vi "CannonProjectileGameFramework.vi"() -> ()   [LabVIEW 2018]
panel:
  out "Distance":dbl
  out "?":cluster{dbl[], dbl[]}(graph)
  out "Score":dbl
  out "Attempt":i32
  out "Wind (mph)":dbl
  out "Target Distance (m)":dbl
  in  "?":bool
  in  "?":bool
  in  "Height (m)":dbl
  in  "Power":dbl
  in  "Angle (deg)":dbl
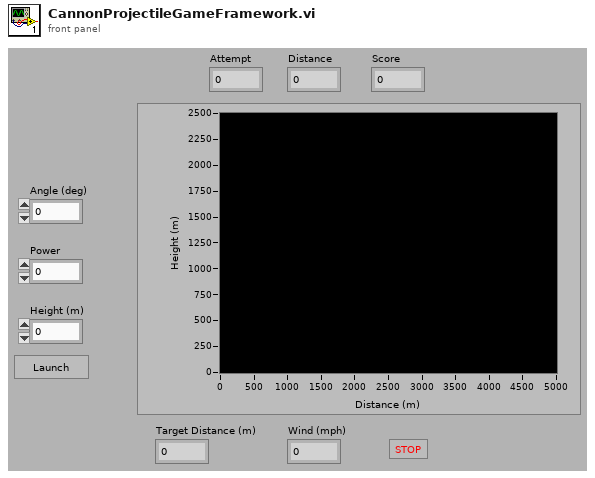
[diagram p1: front panel]
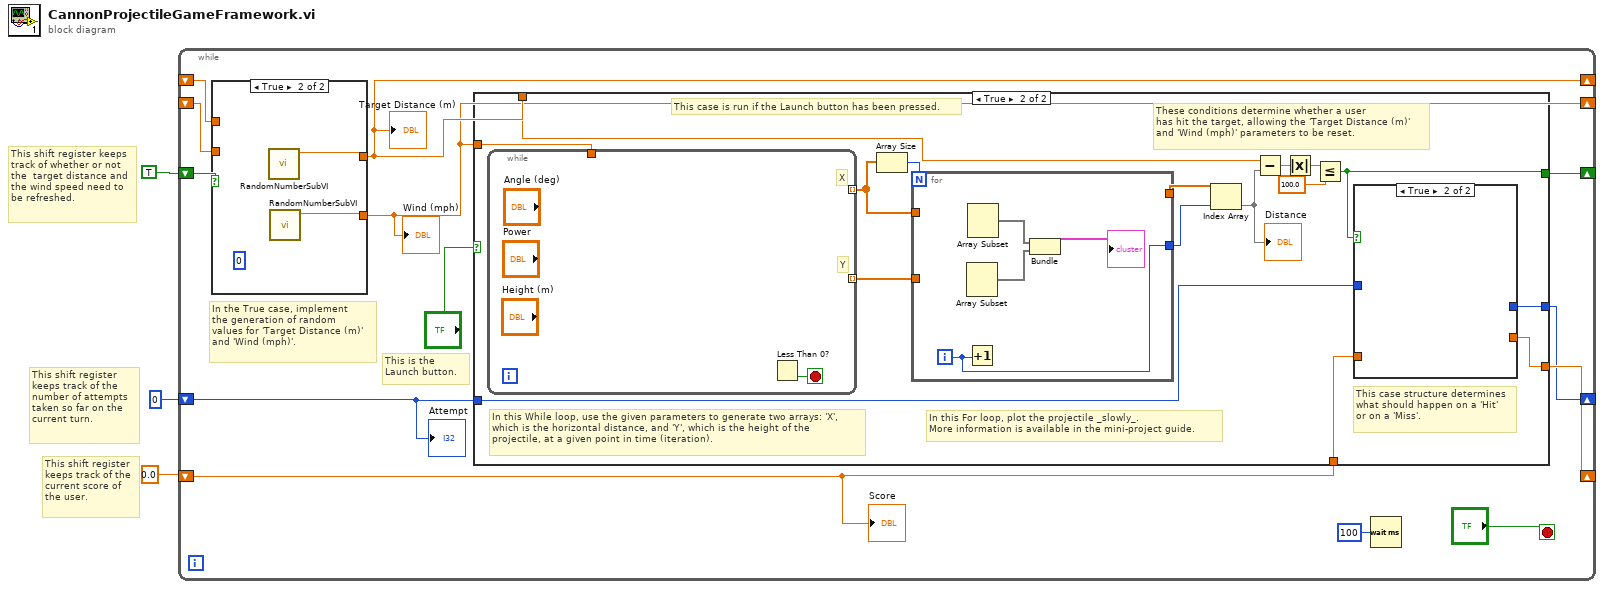
[diagram p0: block diagram]
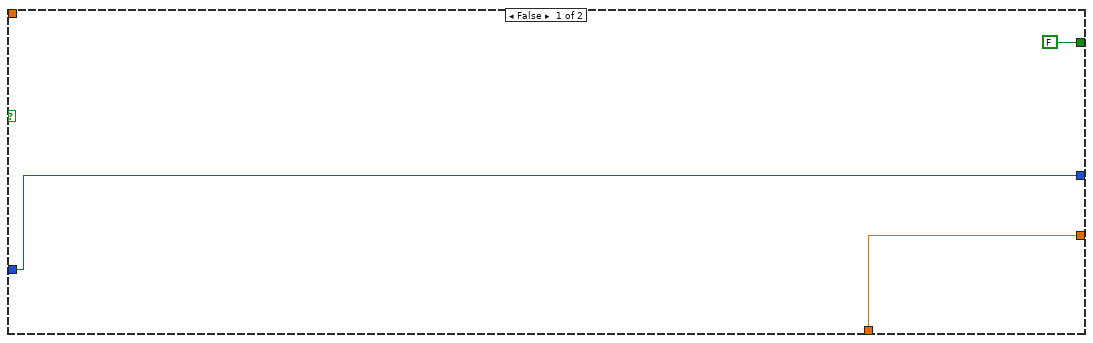
[diagram p3: hidden frame]
diagram:
  # "This shift register keeps\ntrack of whether or not\nthe  target distance and\nthe wind speed need to\nbe refreshed."
  # "This shift register\nkeeps track of the\ncurrent score of\nthe user."
  # "This shift register\nkeeps track of the\nnumber of attempts\ntaken so far on the\ncurrent turn."
  n1 = while {
    shift-right: [w14] -> _
    shift-left: 0.0 -> [w13]
    shift-right: [w12] -> _
    shift-left: 0 -> [w11]
    shift-right: [w9] -> _
    shift-left: TRUE -> [w8]
    shift-right: [w5] -> _
    shift-left: _ -> [w7]
    shift-right: [w4] -> _
    shift-left: _ -> [w6]
    stop <- "?" stop-if-true
    # "This is the Launch button."
    # "In the True case, implement\nthe generation of random\nvalues for 'Target Distance (m)'\nand 'Wind (mph)'."
    n2 = case shown="True" w8 {
      tunnel: [w18 w19] -> w5
      tunnel: [w17 w20] -> w4
      tunnel: w7 -> [w18 _]
      tunnel: w6 -> [w17 _]
      frame False {
      }
      frame True {
        (unwired) 0
        n3 = call "RandomNumberSubVI.vi"() -> ("Random Number"=w19:dbl)  [unwired: 11 in]
        n4 = call "RandomNumberSubVI.vi"() -> ("Random Number"=w20:dbl)  [unwired: 11 in]
      }
    }
    "Target Distance (m)" <- w5
    "Wind (mph)" <- w4
    n5 = case shown="True" "?" {
      tunnel: w5 -> [_ w38]
      tunnel: w4 -> [_ w39]
      tunnel: [w23 w34] -> w12
      tunnel: w11 -> [w23 w25]
      tunnel: [w22 w27] -> w14
      tunnel: w13 -> [w22 w26]
      tunnel: [FALSE w24] -> w9
      frame False {
      }
      frame True {
        # "These conditions determine whether a user\nhas hit the target, allowing the 'Target Distance (m)'\nand 'Wind (mph)' parameters to be reset."
        # "This case is run if the Launch button has been pressed."
        # "This case structure determines\nwhat should happen on a 'Hit'\nor on a 'Miss'."
        # "In this For loop, plot the projectile _slowly_.\nMore information is available in the mini-project guide."
        # "In this While loop, use the given parameters to generate two arrays: 'X',\nwhich is the horizontal distance, and 'Y', which is the height of the\nprojectile, at a given point in time (iteration)."
        n6 = while {
          tunnel: w39 -> [_]
          tunnel: [_] -> w28 mode=indexing
          tunnel: [_] -> w33 mode=indexing
          stop <- w44 stop-if-true
          # "Y"
          # "X"
          n7 = Less Than 0?() -> (x < 0?=w44:bool)  [unwired: 1 in]
        }
        n8 = Array Size(array=w28) -> (size(s)=w29:i32)
        n9 = for {
          N: w29 -> [_]
          tunnel: w28 -> [_]
          tunnel: w33 -> [_]
          tunnel: [_] -> w32
          tunnel: [w41] -> w31
          i -> [w41]
          n10 = Array Subset() -> (w42:void[])  [unwired: 3 in]
          n11 = Increment(x=w41) -> ()  [unwired: 1 out]
          n12 = Array Subset() -> (w43:void[])  [unwired: 3 in]
          n13 = Bundle(w43, w42) -> (→"?":cluster{void[], void[]})  [unwired: 1 out]
        }
        n14 = Index Array(array=w32, index=w31) -> (element=w30)
        "Distance" <- w30
        n15 = Subtract(x=w38, y=w30) -> (x-y=w37:dbl)
        n16 = Absolute Value(x=w37) -> (abs(x)=w36:dbl)
        n17 = Less Or Equal?(x=w36, y=100.0) -> (x <= y?=w24:bool)
        n18 = case shown="True" w24 {
          tunnel: [_ _] -> w34
          tunnel: w25 -> [_ _]
          tunnel: [_ _] -> w27
          tunnel: w26 -> [_ _]
          frame False {
          }
          frame True {
          }
        }
      }
    }
    n19 = Wait (ms)(milliseconds to wait=u32 100) -> ()  [unwired: 1 out]
    "Score" <- w13
    "Attempt" <- w11
  }
